vi "BRAM_ReadAstronaut.vi"(2 "Address":i32) -> (16 "PixelData":bool[](array[boolean]))   [LabVIEW 2018]
uses:
  <vilib>/rvi/Memory/Memory_Emulation/nirvimemoryFastEmulation.vi
  <vilib>/rvi/Memory/Memory_Emulation/nirvimemoryEmulation.vi
  <vilib>/rvi/Emulation/niFpgaEmulationIsFPGAContextNoSignature.vi
  <vilib>/rvi/DataTransferAndStorage/Container/Common/niFpgaContainerGetUniqueNameForEmu.vi
  <vilib>/rvi/Emulation/niFpgaProcessEmulError.vi
  <vilib>/rvi/Emulation/niFpgaSctlEmulationGetInTimedLoop.vi
  <vilib>/rvi/errors/nirviReportUnexpectedCaseInternalError (U32).vi
  <vilib>/rvi/DataTransferAndStorage/Container/XNode/niFpgaContainer.xnode
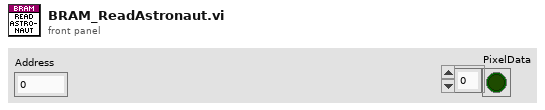
[diagram p1: front panel]
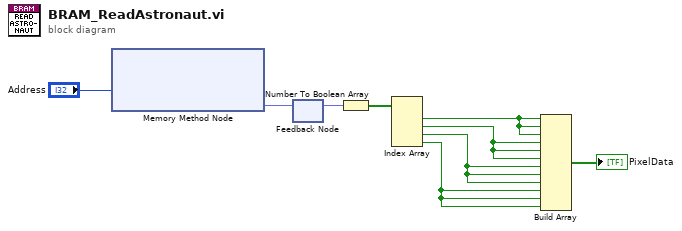
[diagram p0: block diagram]
diagram:
  n1 = xnode ("Memory Method Node")("Address A"="Address") -> ("Data A"=w8:fxp<+,4,4>)  [unwired: 1 in, 1 out]
  n2 = feedback-in #1(w8) -> ()
  n3 = feedback #1() -> (w7:fxp<+,4,4>)  [unwired: 1 in]
  n4 = Number To Boolean Array(number=w7) -> (Boolean array=w2:bool[])
  n5 = Index Array(array=w2) -> (element #1=w3:bool, element #2=w6:bool, element #3=w5:bool, element #4=w4:bool)  [unwired: 4 in]
  n6 = Build Array(w3, w3, w3, w6, w6, w6, w5, w5, w5, w4, w4, w4) -> (→"PixelData":bool[])
